vi "test Check If Custom Device Is Enabled.vi"(8 "error in":errorcluster, 11 "TestCase in":refnum<class "AIM ARINC 664 EncodeDecode.lvclass">) -> (0 "error out":errorcluster, 3 "TestCase out":refnum<class "AIM ARINC 664 EncodeDecode.lvclass">)   [LabVIEW 2020, in "AIM ARINC 664 EncodeDecode.lvclass"]
uses:
  AIM ARINC 664 EncodeDecode.lvclass
  C:/Program Files (x86)/National Instruments/LabVIEW 2020/vi.lib/NI/VeriStand Custom Device Testing Tools/VeriStandScriptingTestCase/VeriStandScriptingTestCase.lvclass
  <vilib>/NI/VeriStand Custom Device Testing Tools/VeriStandScriptingTestCase/VeriStandScriptingTestCase.lvclass/VeriStandScriptingTestCase.ctl
  <vilib>/NI/VeriStand Custom Device Testing Tools/VeriStandScriptingTestCase/Read Target.vi
  NationalInstruments.VeriStand.SystemDefinitionAPI
  <vilib>/addons/_JKI Toolkits/VI Tester/TestCase.llb/TestCase.lvclass
  Scripting/AIM ARINC 664 Scripting.lvlib
  C:/Program Files (x86)/National Instruments/LabVIEW 2020/vi.lib/addons/_JKI Toolkits/VI Tester/TestCase.llb/TestCase.lvclass
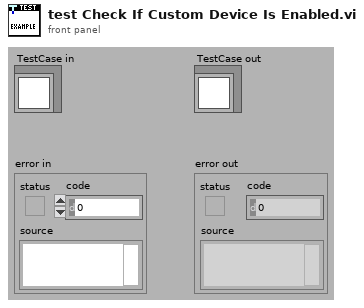
[diagram p1: front panel]
types:
  T1 = typedef "Custom Device API.lvlib/Custom Device Item Ref.ctl" = u64
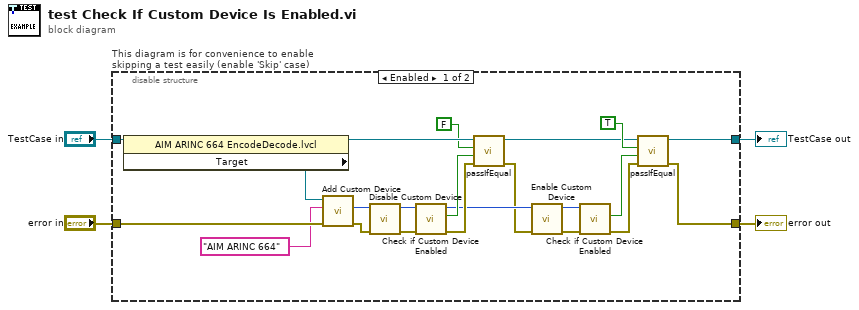
[diagram p0: block diagram]
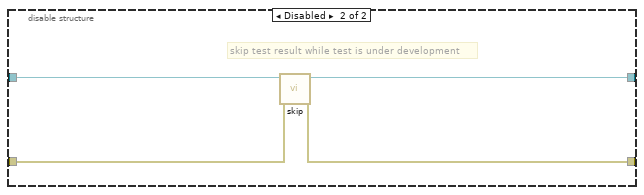
[diagram p2: hidden frame]
diagram:
  n1 = disable-structure "This diagram is for convenience to enable skipping a test easily (enable 'Skip' case)" shown="Enabled" {
    disable-tunnel: "TestCase in" -> [w21 w30]
    disable-tunnel: [w20 w28] -> w1
    disable-tunnel: [w19 w29] -> w3
    disable-tunnel: "error in" -> [w26 w27]
    frame Enabled {
      n2 = property class="AIM ARINC 664 EncodeDecode.lvcl"(reference=w21) -> (reference out=w25:refnum<class "AIM ARINC 664 EncodeDecode.lvclass">, "Target"=w18:refnum<k24>)  [unwired: 1 in, 1 out]
      n3 = call "Add Custom Device.vi"("error in"=w26, "name"="AIM ARINC 664", "target in"=w18) -> ("error out"=w15:errorcluster, "custom device"=w16:T1)  [unwired: 6 in, 1 out]
      n4 = call "Disable Custom Device.vi"("error in"=w15, "custom device ref in"=w16) -> ("error out"=w11:errorcluster, "custom device ref out"=w12:T1)  [unwired: 8 in]
      n5 = call "Check if Custom Device Enabled.vi"("error in"=w11, "custom device ref in"=w12) -> ("error out"=w13:errorcluster, "custom device is enabled"=w14:bool, "custom device ref out"=w10:T1)  [unwired: 7 in]
      n6 = call-dynamic "passIfEqual.vi"("error in (no error)"=w13, "y"=w14, "x"=FALSE ("is enabled?"), "TestCase in"=w25) -> ("error out"=w9:errorcluster, "TestCase out"=w22:refnum<class "AIM ARINC 664 EncodeDecode.lvclass">)  [unwired: 6 in]
      n7 = call "Enable Custom Device.vi"("error in"=w9, "custom device ref in"=w10) -> ("error out"=w5:errorcluster, "custom device ref out"=w6:T1)  [unwired: 8 in]
      n8 = call "Check if Custom Device Enabled.vi"("error in"=w5, "custom device ref in"=w6) -> ("error out"=w8:errorcluster, "custom device is enabled"=w7:bool)  [unwired: 7 in, 1 out]
      n9 = call-dynamic "passIfEqual.vi"("error in (no error)"=w8, "y"=w7, "x"=TRUE ("is enabled?"), "TestCase in"=w22) -> ("error out"=w19:errorcluster, "TestCase out"=w20:refnum<class "AIM ARINC 664 EncodeDecode.lvclass">)  [unwired: 6 in]
    }
    frame Disabled {
      # "skip test result while test is under development"
      n10 = call <vilib>:"skip.vi"("error in (no error)"=w27, "TestCase in"=w30) -> ("error out"=w29:errorcluster, "TestCase out"=w28:refnum<class "AIM ARINC 664 EncodeDecode.lvclass">)  [unwired: 8 in]
    }
  }
  "error out" <- w3
  "TestCase out" <- w1
